vi "NewErrorCode.vi"(8 "ErrorIn":errorcluster caption="Error In(no Error)", 11 "ReferenceIn":refnum<class "ErrorDefinitionSQLite.lvclass"> caption="Reference In") -> (0 "ErrorOut":errorcluster caption="Error Out", 2 "NewErrorCode":i32, 3 "ReferenceOut":refnum<class "ErrorDefinitionSQLite.lvclass"> caption="Reference Out")   [LabVIEW 2018, in "ErrorDefinitionSQLite.lvclass"]
uses:
  <userlib>/_express/CustomErrorCreator/ErrorDefinitionSQLite/ErrorDefinitionSQLite.lvclass
  <vilib>/drjdpowell/SQLite Library/SQL Connection/Open (path).vi
  <vilib>/drjdpowell/SQLite Library/SQL Connection/Open (string).vi
  <vilib>/AdvancedString/Path To Command Line String.vi
  <vilib>/drjdpowell/SQLite Library/SQL Connection/Execute SQL.vi
  <vilib>/drjdpowell/SQLite Library/SQL Connection/Connection.lvclass
  <vilib>/drjdpowell/SQLite Library/Transaction Helpers/Transaction.lvlib
  <vilib>/drjdpowell/SQLite Library/SQLite.lvlib
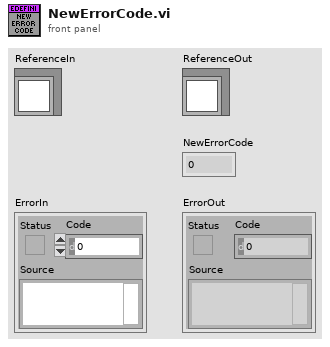
[diagram p1: front panel]
types:
  T1 = enum16{"New or existing", "Existing", "Read only"}
  T2 = typedef "ErrorDefinitionSQLite.lvclass/ObjectAttributes.ctl" = cluster{"Path":path}
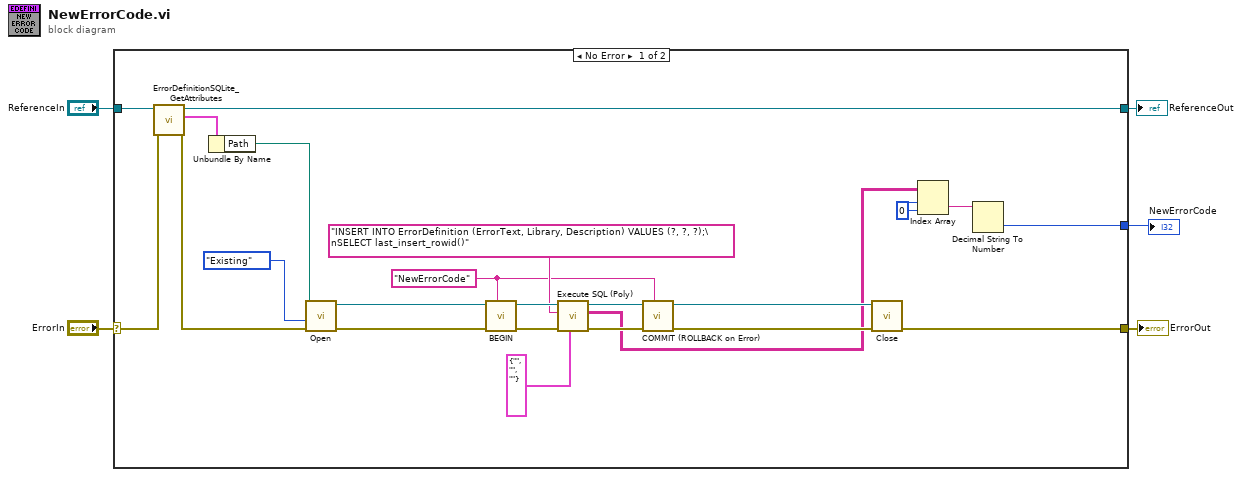
[diagram p0: block diagram]
diagram:
  n1 = case shown="No Error" "ErrorIn" {
    selector: "ErrorIn" -> [w28 w30]
    tunnel: [w21 w30] -> w4
    tunnel: [w26 w29] -> w2
    tunnel: "ReferenceIn" -> [w27 w29]
    tunnel: [w6 _] -> w1
    frame No Error {
      w11 = "NewErrorCode" ("Savepoint name")
      w7 = 0 ("disabled index (col)")
      n2 = call <userlib>:"ErrorDefinitionSQLite_GetAttributes.vi"("ErrorIn"=w28, "Reference in"=w27) -> ("ErrorOut"=w22:errorcluster, "Data"=w24:T2, "Reference out"=w26:refnum<class "ErrorDefinitionSQLite.lvclass">)  [unwired: 6 in, 1 out]
      n3 = Unbundle By Name(w24) -> ("Path"=w23:path)
      n4 = call-poly <vilib>:"Open.vi"("error in (no error)"=w22, "File Option"=T1."Existing", "db file"=w23) -> ("error out"=w16:errorcluster, "SQLite Connection"=w15:refnum<class "Connection.lvclass">)  [unwired: 7 in]
      n5 = call <vilib>:"BEGIN.vi"("Savepoint name"=w11, "error in (no error)"=w16, "SQLite Connection in"=w15) -> ("error out"=w18:errorcluster, "SQLite Connection"=w19:refnum<class "Connection.lvclass">)  [unwired: 7 in]
      n6 = call-poly <vilib>:"Execute SQL (Poly).vi"("Parameter(s)"=cluster{string, string, string} {"", "", ""}, "error in (no error)"=w18, "SQL"="INSERT INTO ErrorDefinition (ErrorText, Library, Description) VALUES (?, ?, ?);\nSELECT last_insert_rowid()", "SQLite Connection in"=w19) -> ("error out"=w13:errorcluster, "Result Set"=w8:string[][], "SQLite Connection"=w12:refnum<class "Connection.lvclass">)  [unwired: 4 in, 1 out]
      n7 = call <vilib>:"COMMIT (ROLLBACK on Error).vi"("Savepoint name"=w11, "error in (no error)"=w13, "SQLite Connection in"=w12) -> ("error out"=w10:errorcluster, "SQLite Connection"=w9:refnum<class "Connection.lvclass">)  [unwired: 7 in]
      n8 = call-dynamic "Close.vi"("error in (no error)"=w10, "SQLite Connection in"=w9) -> ("error out"=w21:errorcluster)  [unwired: 9 in]
      n9 = Index Array(array=w8, index (row)=w7, index (col)=w7) -> (element=w20:string)
      n10 = Decimal String To Number(string=w20) -> (number=w6:i32)  [unwired: 2 in, 1 out]
    }
    frame Error {
    }
  }
  "ErrorOut" <- w4
  "ReferenceOut" <- w2
  "NewErrorCode" <- w1
